vi "Thermal Camera 1.vi"() -> ()   [LabVIEW 2025]
uses:
  libirimager-8.9.0-windows/irDirectSDK/examples/labview/libirimager_direct_binding.lvlib
panel:
  in  "Stop":bool
  out "function return 2":i32
  out "H out":i32
  out "W out":i32
  in  "xml_camera_config":string
  in  "Start Feed":bool
  in  "Connect USB":bool
  out "new picture":picture
  out "thermal_data out":u16[](array[numeric])
  out "function return thm":i32
  out "w out":i32
  out "h out":i32
  out "function return save png":i32
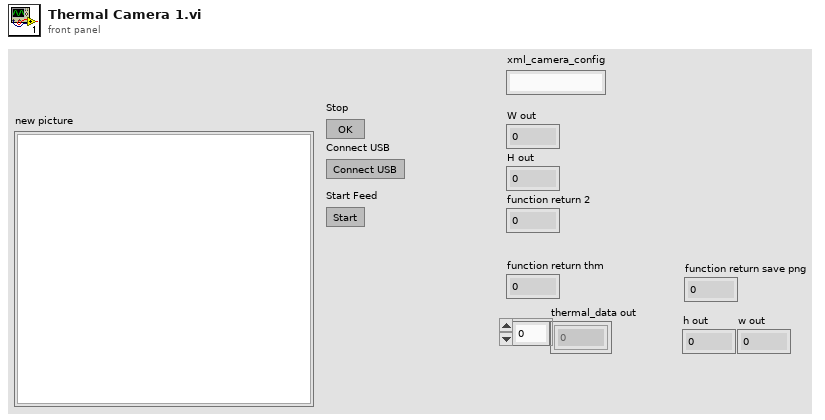
[diagram p1: front panel]
types:
  T1 = typedef "imagedata.ctl" = cluster{"image type":i32, "image depth":i32, "image":u8[], "mask":u8[], "colors":u32[], "Rectangle":cluster{"left":i16, "top":i16, "right":i16, "bottom":i16}}
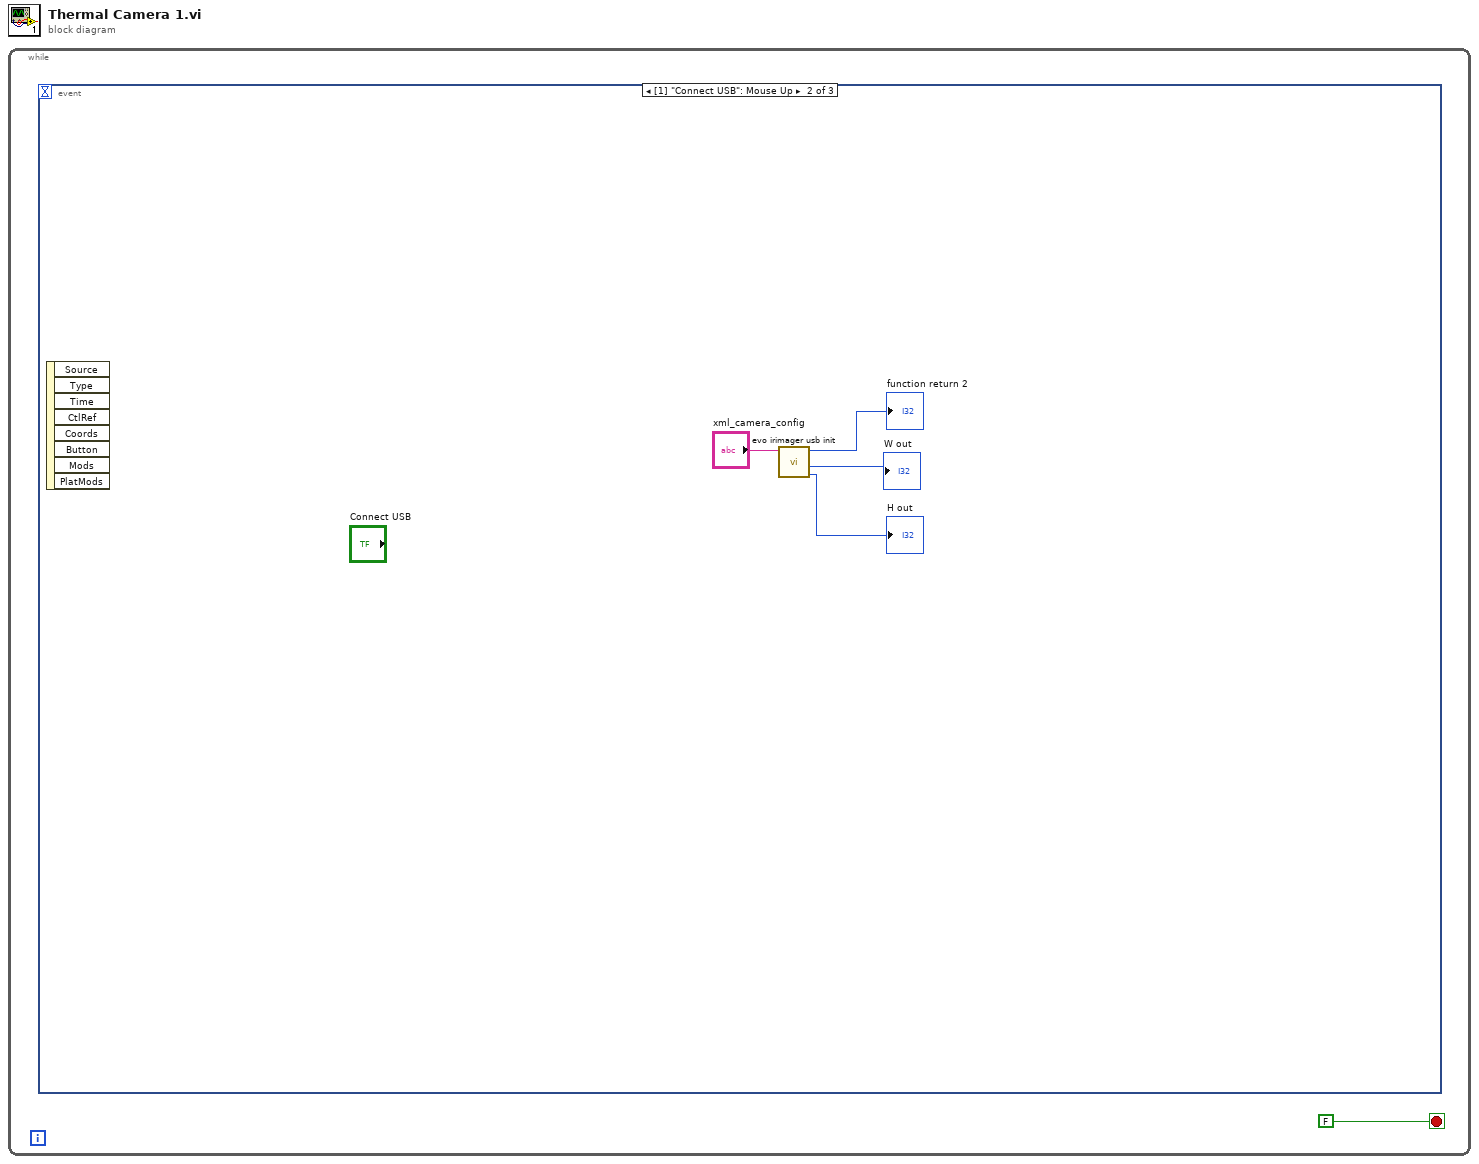
[diagram p0: block diagram]
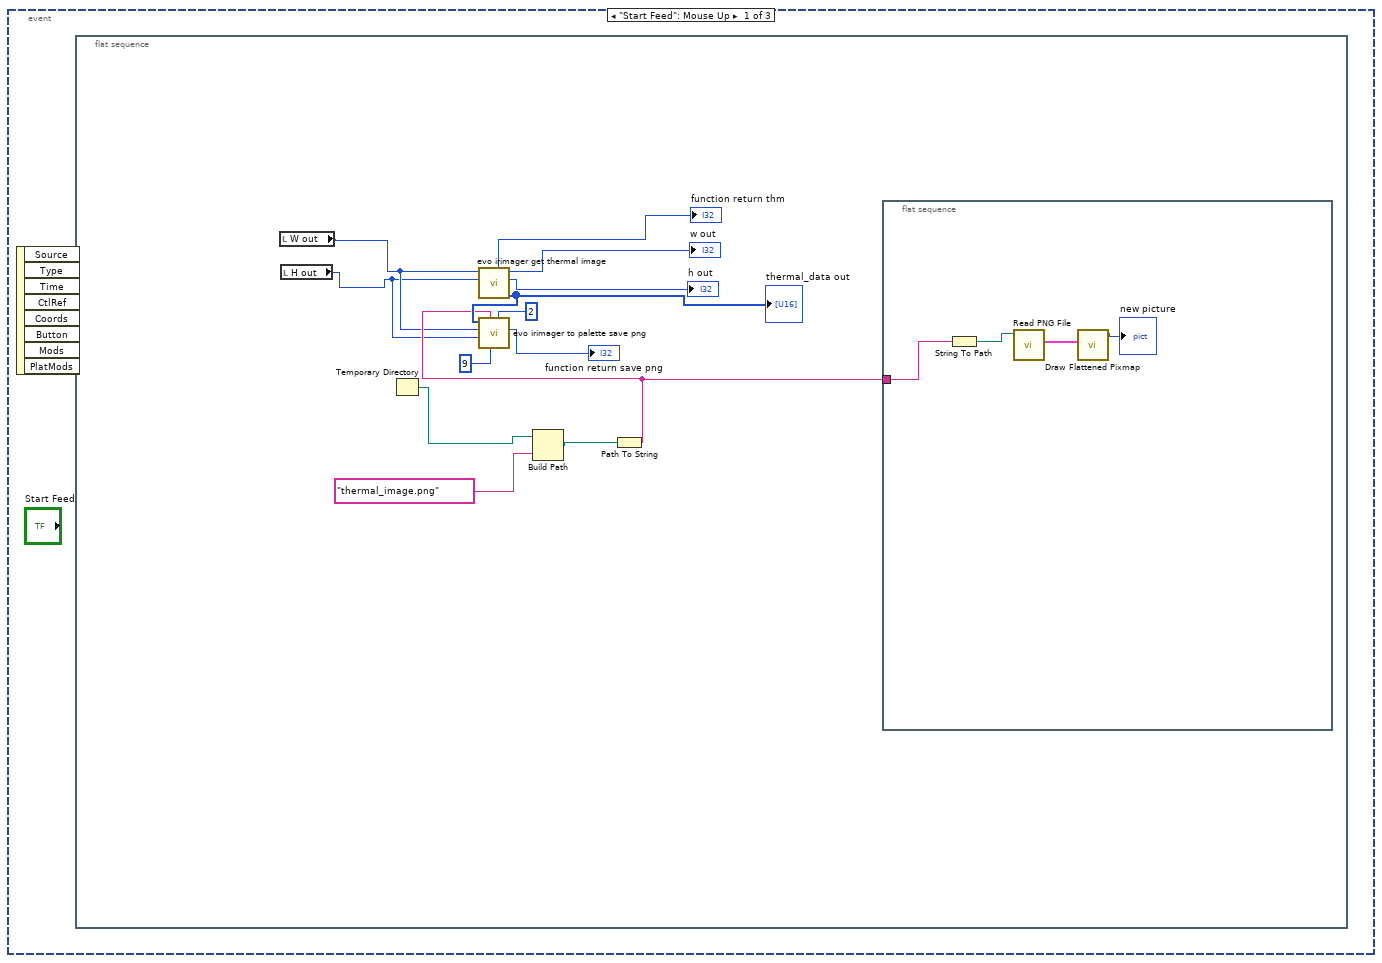
[diagram p2: hidden frame]
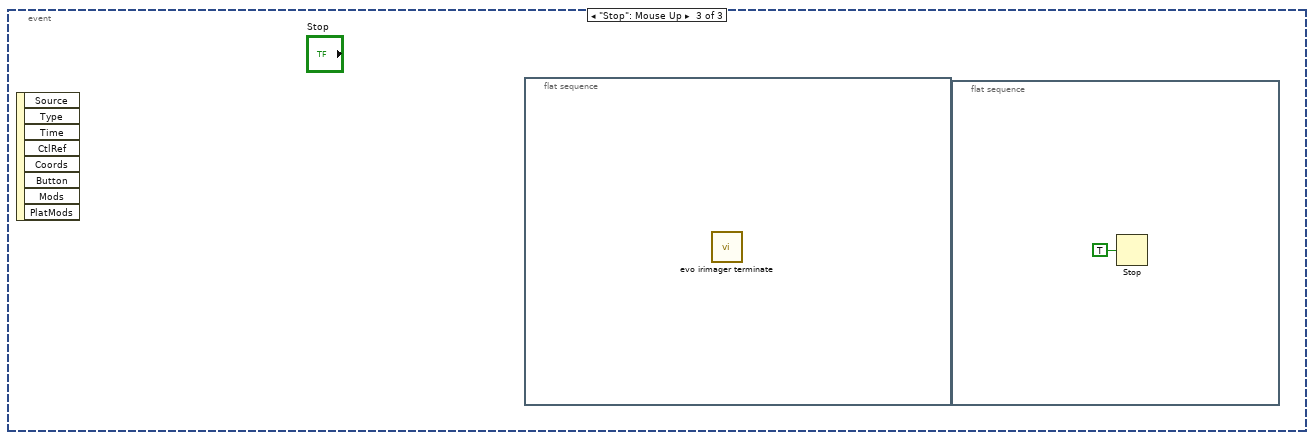
[diagram p3: hidden frame]
diagram:
  n1 = while {
    stop <- FALSE stop-if-true
    n2 = event shown="[1] \"Connect USB\": Mouse Up" {
      selector: _ -> [_ _ _]
      dyn-events: _ -> [_ _ _]
      timeout: _ -> [_ _ _]
      event "Start Feed": Mouse Up {
        n3 = event-data() -> ()  [unwired: 1 in, 8 out]
        n4 = flat-sequence {
          frame #0 {
            n5 = local read "W out"() -> (w3:i32)
            n6 = local read "H out"() -> (w2:i32)
            n7 = Temporary Directory() -> (w6:path)
            n8 = call "evo irimager get thermal image.vi"("h"=w2, "w"=w3) -> ("data out"=w8:u16[], "h out"=→"h out":i32, "w out"=→"w out":i32, "function return"=→"function return thm":i32)  [unwired: 6 in]
            "thermal_data out" <- w8
            n9 = Build Path(base path=w6, name or relative path="thermal_image.png" ("String")) -> (appended path=w5:path)
            n10 = Path To String(path=w5) -> (string=w4:string)
            n11 = call "evo irimager to palette save png.vi"("palette_scale"=2, "palette"=9, "path"=w4, "h"=w2, "w"=w3, "thermal_data"=w8) -> ("function return"=→"function return save png":i32)  [unwired: 4 in, 1 out]
            n12 = flat-sequence {
              tunnel: w4 -> [w18]
              frame #0 {
                n13 = String To Path(string=w18) -> (path=w17:path)
                n14 = call <vilib>:"Read PNG File.vi"("path to PNG file"=w17) -> ("image data"=w16:T1)  [unwired: 8 in, 2 out]
                n15 = call <vilib>:"Draw Flattened Pixmap.vi"("image data"=w16) -> ("new picture"=→"new picture":picture)  [unwired: 8 in]
              }
            }
          }
        }
      }
      event "Connect USB": Mouse Up {
        n16 = event-data() -> ()  [unwired: 1 in, 8 out]
        n17 = call "evo irimager usb init.vi"("xml_config"="xml_camera_config") -> ("h out"=→"H out":i32, "w out"=→"W out":i32, "function return 2"=→"function return 2":i32)  [unwired: 7 in, 1 out]
      }
      event "Stop": Mouse Up {
        n18 = event-data() -> ()  [unwired: 1 in, 8 out]
        n19 = flat-sequence {
          frame #0 {
            n20 = call "evo irimager terminate.vi"() -> ()  [unwired: 11 in, 1 out]
          }
        }
        n21 = flat-sequence {
          frame #0 {
            n22 = Stop(stop? (T)=TRUE ("Stopp? (T)")) -> ()
          }
        }
      }
    }
  }
